vi "Init.vi"(8 "error in (no error)":errorcluster) -> (0 "error out":errorcluster, 3 "Model out":refnum<class "Model.lvclass">)   [LabVIEW 2020, in "Model.lvlib" / "Model.lvclass"]
uses:
  Model.lvclass
  Model.lvclass/Model.ctl
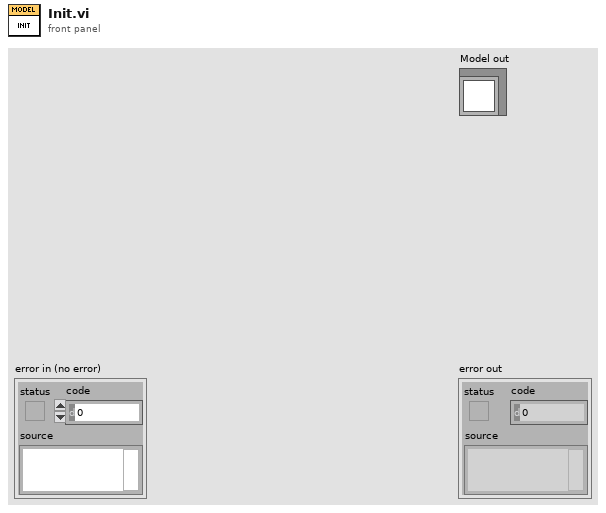
[diagram p1: front panel]
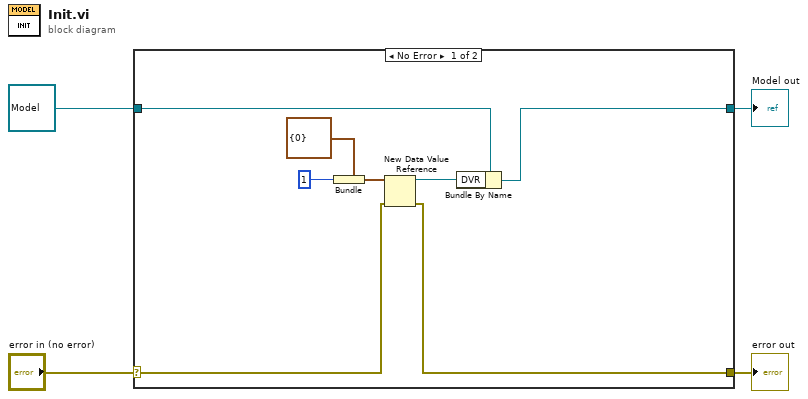
[diagram p0: block diagram]
diagram:
  n1 = case shown="No Error" "error in (no error)" {
    selector: "error in (no error)" -> [w6 w14]
    tunnel: [w5 w14] -> w3
    tunnel: [w9 w13] -> w2
    tunnel: refnum<class "Model.lvclass"> refnum ("Model in") -> [w10 w13]
    frame No Error {
      n2 = Bundle(cluster=cluster{"Integer":i32} {"Integer"=0} ("output cluster"), "Integer"=1) -> (w11:cluster{"Integer":i32})
      n3 = New Data Value Reference(data value=w11, error in=w6) -> (data value reference=w7:refnum<data-value>, error out=w5:errorcluster)
      n4 = Bundle By Name(cluster=w10, "DVR"=w7) -> (w9:refnum<class "Model.lvclass">)
    }
    frame Error {
    }
  }
  "error out" <- w3
  "Model out" <- w2
